vi "Create All Message Queues.vi"(8 "error in (no error)":errorcluster) -> (0 "error out":errorcluster, 3 "Message Queues out":T1)   [LabVIEW 2024, in "Message Queue.lvlib"]
doc: "This VI creates and initializes all the message queues for your application. If your application requires more than one message queue, right-click the \"Message Queues\" constant above and select Open Type Def. Add the new Message Queue(s) to the type definition, then initialize them in this VI."
uses:
  Message Queue.lvlib
  All Message Queues.ctl
  Message Cluster.ctl
  Enqueue Message (Single).vi
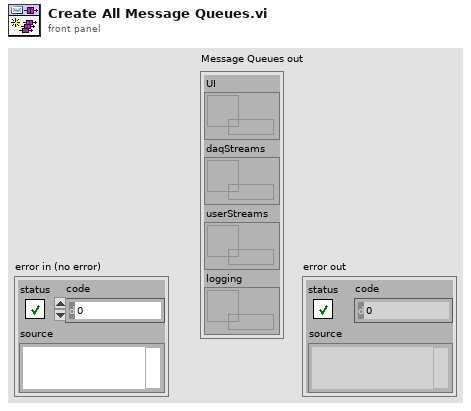
[diagram p1: front panel]
types:
  T1 = typedef "Message Queue.lvlib/All Message Queues.ctl" = cluster{"UI":refnum<queue>, "daqStreams":refnum<queue>, "userStreams":refnum<queue>, "logging":refnum<queue>}
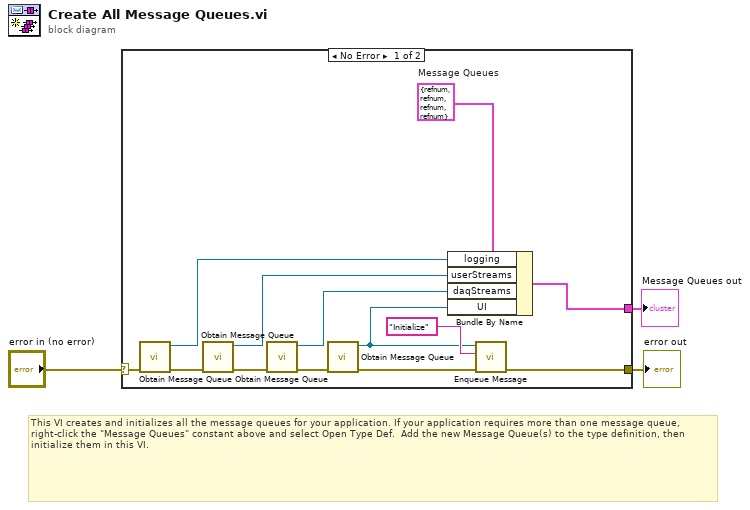
[diagram p0: block diagram]
diagram:
  # "This VI creates and initializes all the message queues for your application. If your application requires more than one message queue, right-click the \"Message Queues\" constant above and select Open Type Def.  Add the new Message Queue(s) to the type definition, then initialize them in this VI."
  n1 = case shown="No Error" "error in (no error)" {
    selector: "error in (no error)" -> [w10 w17]
    tunnel: [w16 w17] -> w3
    tunnel: [w14 _] -> w2
    frame No Error {
      w15 = T1 {"UI"=refnum, "daqStreams"=refnum, "userStreams"=refnum, "logging"=refnum}  # Message Queues
      n2 = call "Obtain Message Queue.vi"("error in (no error)"=w10) -> ("error out"=w9:errorcluster, "Message Queue"=w4:refnum<queue>)  [unwired: 9 in]
      n3 = call "Obtain Message Queue.vi"("error in (no error)"=w9) -> ("error out"=w8:errorcluster, "Message Queue"=w5:refnum<queue>)  [unwired: 9 in]
      n4 = call "Obtain Message Queue.vi"("error in (no error)"=w8) -> ("error out"=w7:errorcluster, "Message Queue"=w6:refnum<queue>)  [unwired: 9 in]
      n5 = call "Obtain Message Queue.vi"("error in (no error)"=w7) -> ("error out"=w13:errorcluster, "Message Queue"=w11:refnum<queue>)  [unwired: 9 in]
      n6 = Bundle By Name(cluster=w15, "logging"=w4, "userStreams"=w5, "daqStreams"=w6, "UI"=w11) -> (w14:T1)
      n7 = call-poly "Enqueue Message.vi"("error in (no error)"=w13, "Message"="Initialize", "Message Queue"=w11) -> ("error out"=w16:errorcluster)  [unwired: 7 in, 1 out]
    }
    frame Error {
    }
  }
  "Message Queues out" <- w2
  "error out" <- w3
